vi "channeldata_2ch_complexbigendianinterleaved.vi"() -> ()   [LabVIEW 2019]
panel:
  out "Error Out":errorcluster
  in  "TDMS File":path=path "C:/Python/projects/nitdms/tests/tdms_files/channeldata_2ch_complexbigendianinterleaved.tdms"
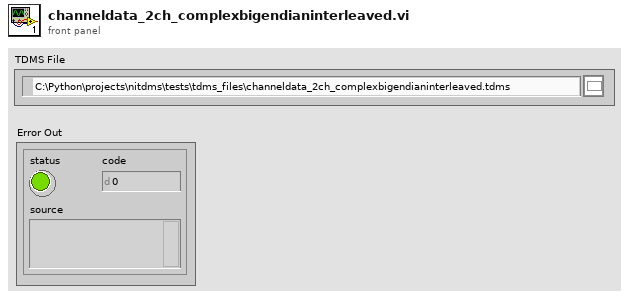
[diagram p1: front panel]
types:
  T1 = enum16{"big-endian, network order", "native, host order", "little-endian"}
  T2 = enum16{"open", "open or create", "create or replace", "create", "open (read-only)"}
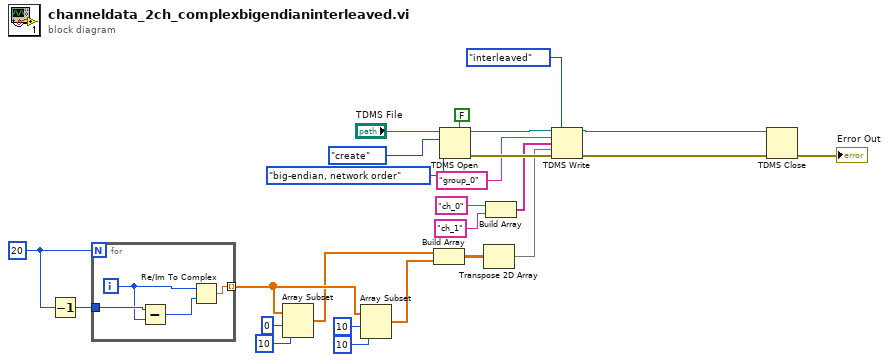
[diagram p0: block diagram]
diagram:
  w2 = 20
  n1 = Decrement(x=w2) -> (x-1=w1:i32)
  n2 = for {
    N: w2 -> [_]
    tunnel: [w26] -> w14 mode=indexing
    tunnel: w1 -> [w29]
    i -> [w28]
    n3 = Subtract(x=w29, y=w28) -> (x-y=w27:i32)
    n4 = Re/Im To Complex(1:w27, 2:w28) -> (0:w26:cdb)
  }
  n5 = Array Subset(array=w14, index=0, length=10) -> (w13:cdb[])
  n6 = Array Subset(array=w14, index=10, length=10) -> (w12:cdb[])
  n7 = Build Array(w13, w12) -> (w5:cdb[][])
  n8 = TDMS Open(5:FALSE ("create index file? (T)"), 9:T1."big-endian, network order" ("byte order (2:little-endian)"), 10:T2."create" ("operation (0:open)"), 11:"TDMS File") -> (0:w21:errorcluster, 3:w20:refnum<k34>)  [unwired: 3 in]
  n9 = Transpose 2D Array(2D array=w5) -> (transposed array=w4:cdb[][])
  n10 = Build Array("ch_0", "ch_1") -> (w9:string[])
  n11 = TDMS Write(0:w20, 1:enum16{"decimated", "interleaved"}."interleaved" ("data layout (0:decimated)"), 5:"group_0", 7:w9, 9:w4, 11:w21) -> (4:w7:refnum<k34>, 15:w8:errorcluster)  [unwired: 2 out]
  n12 = TDMS Close(8:w8, 11:w7) -> (0:→"Error Out":errorcluster)  [unwired: 1 out]
